vi "主画面.vi"() -> ()   [LabVIEW 2016]
uses:
  <vilib>/Utility/miscctls.llb/LVPointTypeDef.ctl
  <vilib>/Averna/Notify Icon/NotifyIcon.llb/BalloonIcon.ctl
  <vilib>/Utility/config.llb/Write Key (String).vi
  <vilib>/Utility/config.llb/Write Key (U32).vi
  <vilib>/Utility/config.llb/Read Key (String).vi
  <vilib>/Utility/config.llb/Read Key (I32).vi
  <vilib>/Averna/Notify Icon/NotifyIcon.llb/GetSelectedItemEvent.vi
  <vilib>/Averna/Notify Icon/NotifyIcon.llb/SetVisible.vi
  <vilib>/Averna/Notify Icon/NotifyIcon.llb/SetMenuDefaultItem.vi
  <vilib>/Averna/Notify Icon/NotifyIcon.llb/SetTipText.vi
  <vilib>/FTP/NI_FTP.lvlib
  <vilib>/Averna/Notify Icon/NotifyIcon.llb/NotifyIcon.lvclass
  <vilib>/Utility/config.llb/NI_LVConfig.lvlib
panel:
  in  "AniGIF":refnum<k7>(container)
  in  "TCP数据输入":string
  in  "开机启动":bool
  in  "超时毫秒(25000)":i32
  in  "模式（标准）":T1(ring)
  out "error out":errorcluster
  in  "停止":bool
  out "程序更新次数":i32
  out "错误TCP":errorcluster caption="错误输出"
  out "连接ID":refnum<k5>
  in  "远程端口或服务名称":u16=1000
  in  "地址":string="127.0.0.1"
  out "当前状态":enum16{"open", "read", "write", "close"}(ring)
  out "通讯":bool
  out "心跳包计数":i32
  out "TCP数据读取":string
  in  "流程启动":bool
  in  "QN":string
  out "日期/时间字符串":string
  out "步骤":string
  out "流程信息":string
  in  "local path":path=path "C:/Users/Administrator/Desktop/ftp接收文件/一体化微型水质监测站.exe"
  in  "filename":string="一体化微型水质监测站.exe"
  in  "passWord":string="std23506"
  in  "userName":string="cc"
  in  "address":string="192.168.16.237"
  # "examples:\nftp.ni.com\nftp.kernel.org\nftp.microsoft.com"
  # "从TCP端读取的信息有：\n1.FTP的address\n2.username\n3.password\n4.filename(.exe)\n5.local path"
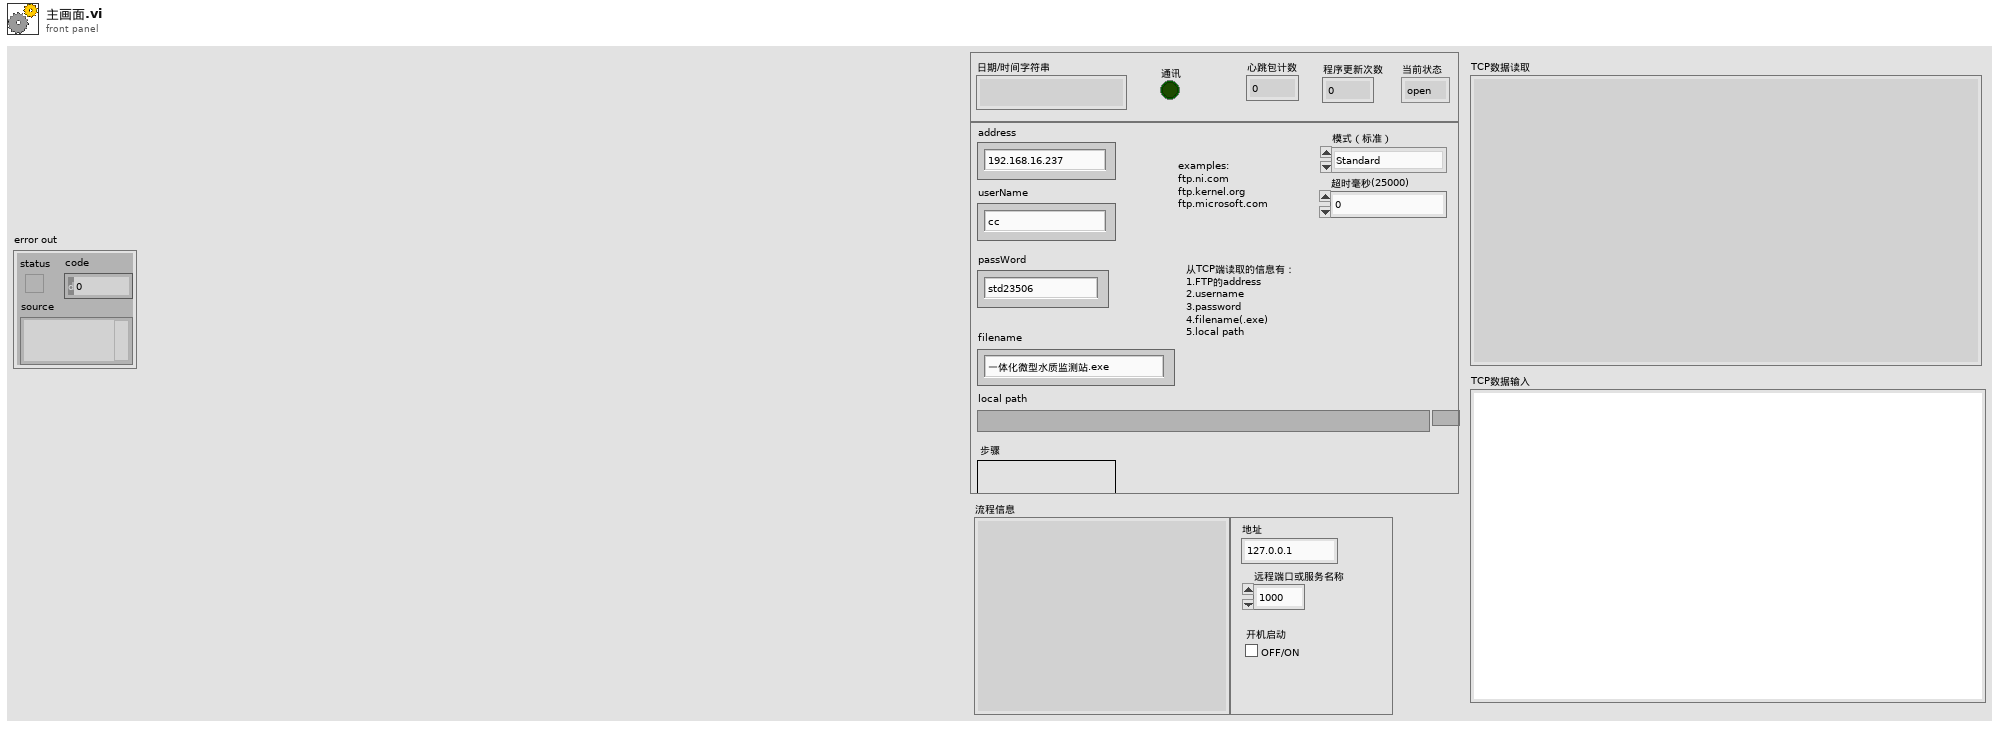
[diagram p1: front panel]
types:
  T1 = enum16{"Standard", "Buffered", "CRLF", "Immediate"}
  T2 = typedef "LVPointTypeDef.ctl" = cluster{"Horizontal":i16, "Vertical":i16}
  T3 = typedef "NI_LVConfig.lvlib/Config Data RefNum.ctl" = refnum<k1>
  T4 = enum32{"invalid app kind", "Development System", "Run Time System", "Student Edition", "Embedded LabVIEW", "Evaluation", "Custom"}
  T5 = enum32{"Invalid", "Standard", "Closed", "Hidden", "Minimized", "Maximized"}
  T6 = enum16{"init", "download", "close", "replace", "open", "over"}
  T7 = typedef "NotifyIcon.lvlib/NotifyIcon.lvclass/BalloonIcon.ctl" = enum32{"None", "Information", "Warning", "Error"}
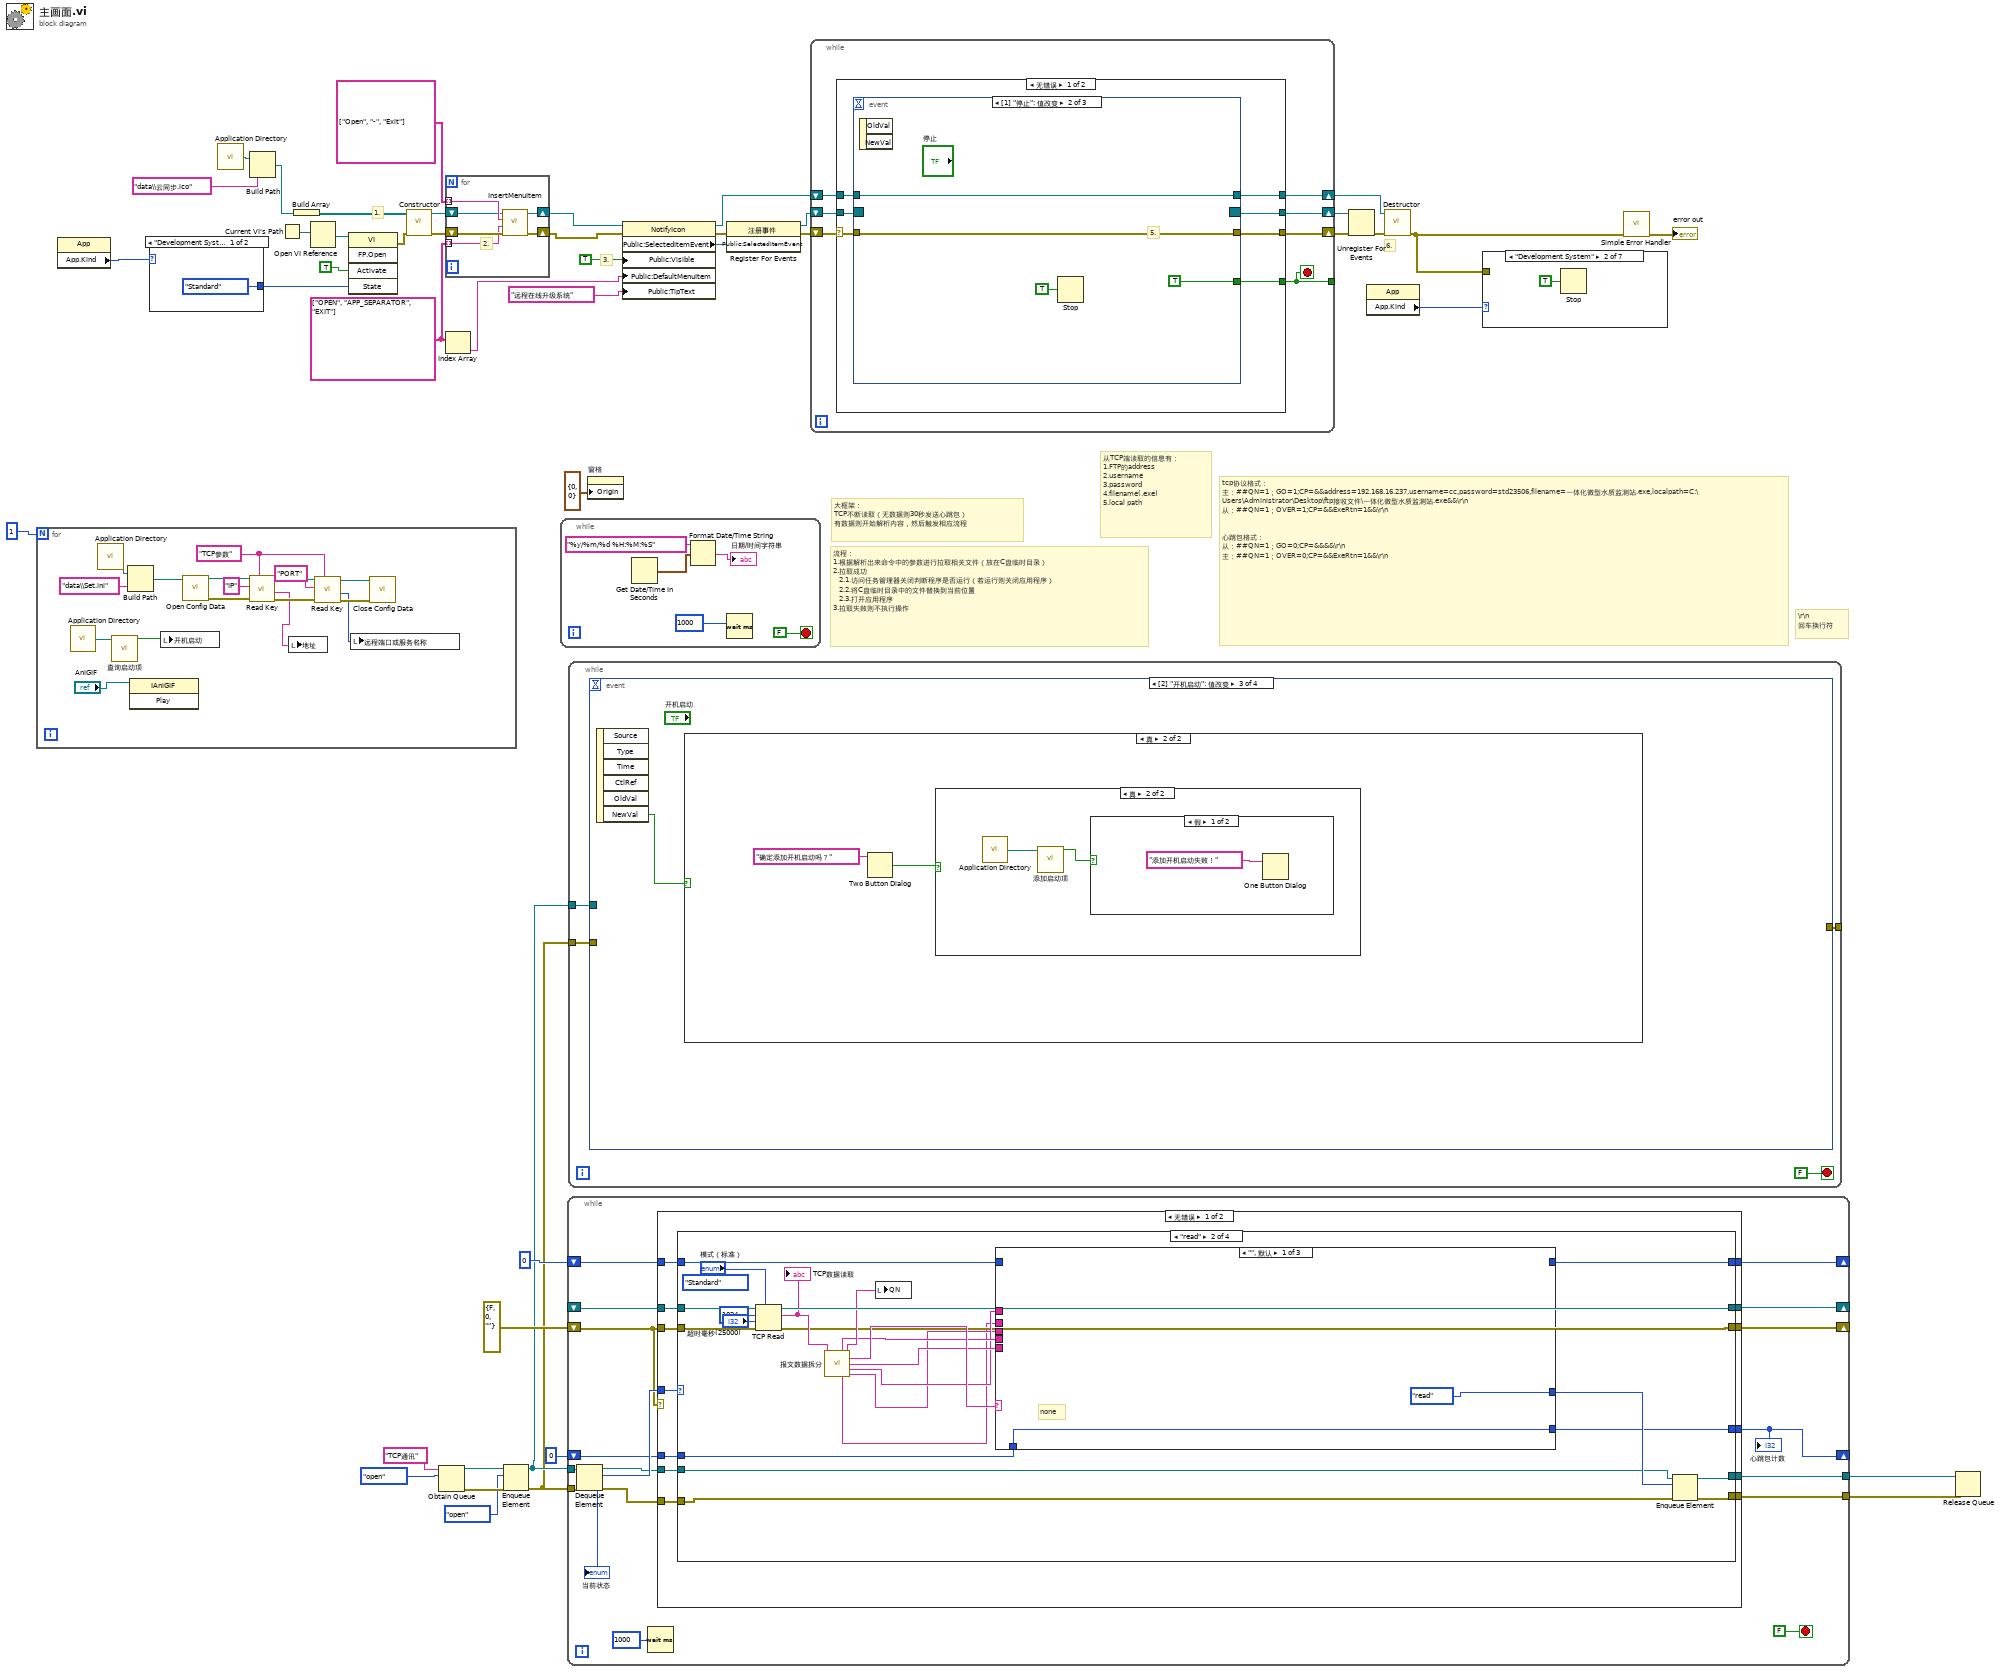
[diagram p0: block diagram]
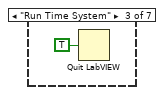
[diagram p3: hidden frame]
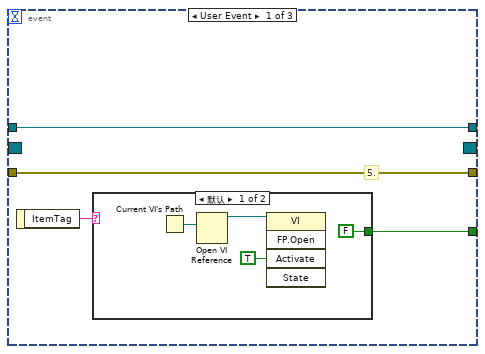
[diagram p8: hidden frame]
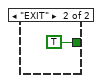
[diagram p9: hidden frame]
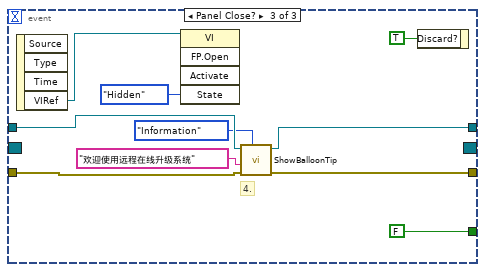
[diagram p10: hidden frame]
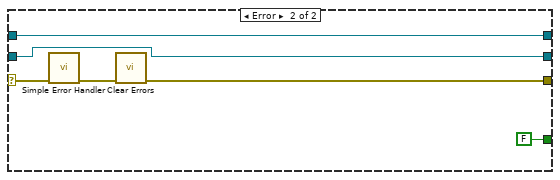
[diagram p11: hidden frame]
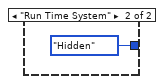
[diagram p12: hidden frame]
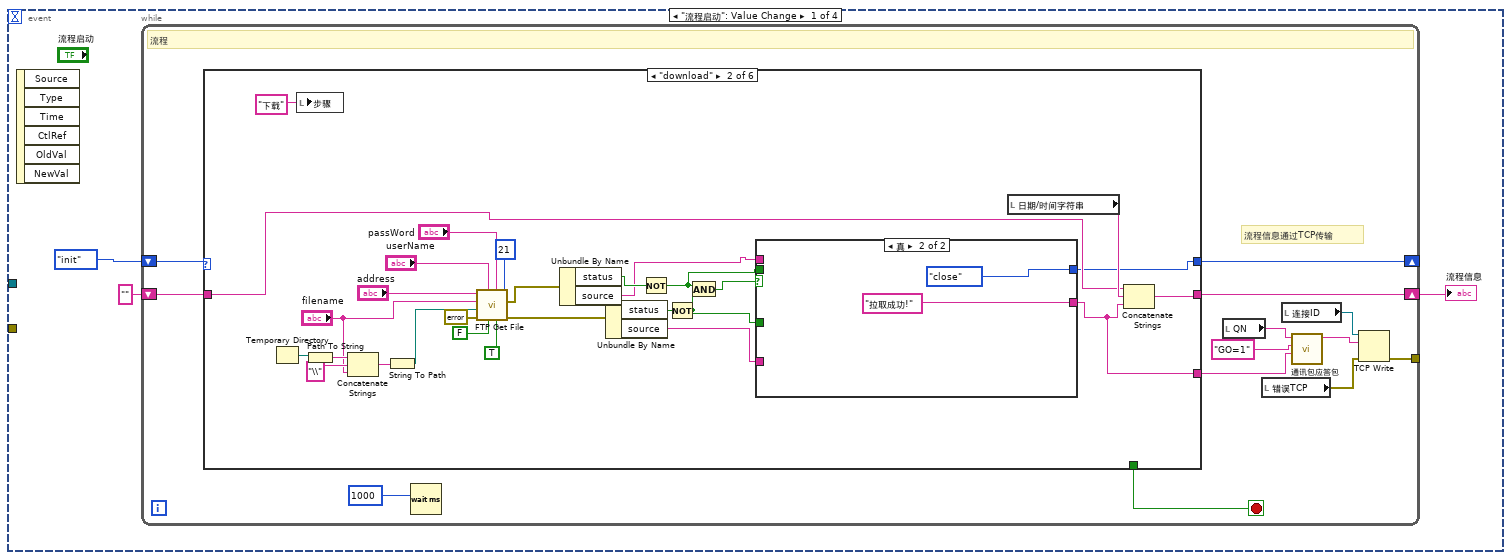
[diagram p13: hidden frame]
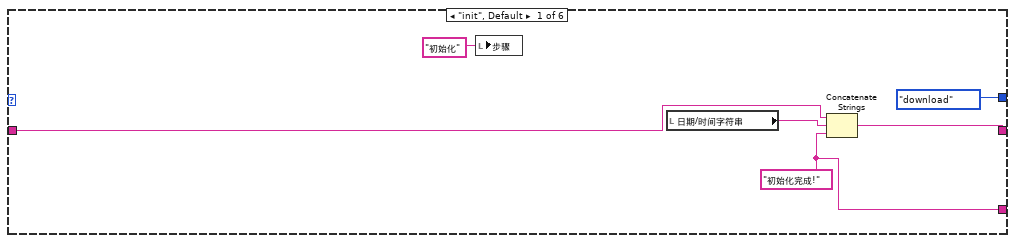
[diagram p14: hidden frame]
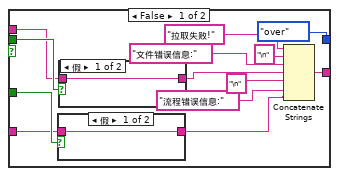
[diagram p15: hidden frame]
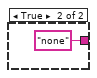
[diagram p16: hidden frame]
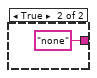
[diagram p17: hidden frame]
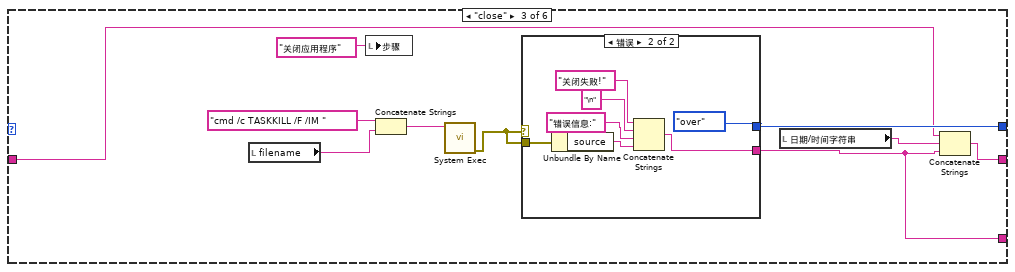
[diagram p18: hidden frame]
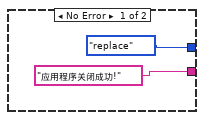
[diagram p19: hidden frame]
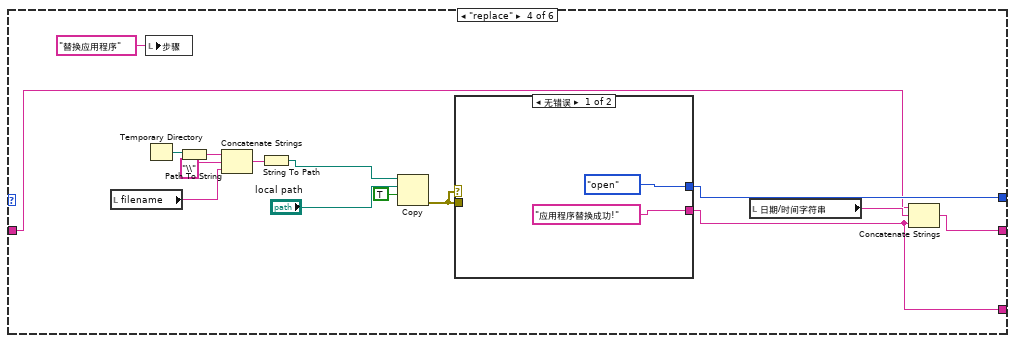
[diagram p20: hidden frame]
diagram:
  w24 = string[] ["OPEN", "APP_SEPARATOR", "EXIT"]
  # "6."
  # "3."
  # "1."
  # "\\r\\n\n回车换行符"
  # "tcp协议格式：\n主：##QN=1；GO=1;CP=&&address=192.168.16.237,username=cc,password=std23506,filename=一体化微型水质监测站.exe,localpath=C:\\Users\\Administrator\\Desktop\\ftp接收文件\\一体化微型水质监测站.exe&&\\r\\n\n从：##QN=1；OVER=1;CP=&&ExeRtn=1&&\\r\\n\n\n\n心跳包格式：\n从：##QN=1；GO=0;CP=&&&&\\r\\n\n主：##QN=1；OVER=0;CP=&&ExeRtn=1&&\\r\\n"
  # "从TCP端读取的信息有：\n1.FTP的address\n2.username\n3.password\n4.filename(.exe)\n5.local path"
  # "流程：\n1.根据解析出来命令中的参数进行拉取相关文件（放在C盘临时目录）\n2.拉取成功\n   2.1.访问任务管理器关闭判断程序是否运行（若运行则关闭应用程序）\n   2.2.将C盘临时目录中的文件替换到当前位置\n   2.3.打开应用程序\n3.拉取失败则不执行操作"
  # "大框架：\nTCP不断读取（无数据则30秒发送心跳包）\n有数据则开始解析内容，然后触发相应流程"
  n1 = for {
    N: 1 -> [_]
    w52 = "TCP参数" ("section")
    n2 = call <vilib>:"Application Directory.vi"() -> ("Application Directory"=w48:path)
    n3 = call <vilib>:"Application Directory.vi"() -> ("Application Directory"=w60:path)
    n4 = call "查询启动项.vi"("启动文件路径"=w48) -> ("包含启动项"=w47:bool)  [unwired: 9 in, 1 out]
    n5 = Build Path(base path=w60, name or relative path="data\\Set.ini" ("名称或相对路径")) -> (appended path=w58:path)
    n6 = invoke class="IAniGIF" method="Play"(reference="AniGIF") -> ()  [unwired: 2 in, 3 out]
    n7 = local write "开机启动"(w47) -> ()
    n8 = call <vilib>:"Open Config Data.vi"("configuration file path"=w58) -> ("error out"=w61:errorcluster, "refnum"=w62:T3)  [unwired: 8 in, 1 out]
    n9 = call-poly <vilib>:"Read Key.vi"("section"=w52, "error in (no error)"=w61, "key"="IP", "refnum"=w62) -> ("error out"=w56:errorcluster, "value"=w50:string, "refnum out"=w57:T3)  [unwired: 4 in, 1 out]
    n10 = local write "地址"(w50) -> ()
    n11 = call-poly <vilib>:"Read Key.vi"("section"=w52, "error in (no error)"=w56, "key"="PORT", "refnum"=w57) -> ("error out"=w54:errorcluster, "value"=w49:i32, "refnum out"=w55:T3)  [unwired: 4 in, 1 out]
    n12 = local write "远程端口或服务名称"(w49) -> ()
    n13 = call <vilib>:"Close Config Data.vi"("error in (no error)"=w54, "refnum"=w55) -> ()  [unwired: 8 in, 2 out]
  }
  n14 = property class="App"() -> ("App.Kind"=w32:T4)  [unwired: 2 in, 2 out]
  n15 = case shown="\"Development System\", 默认" w32 {
    tunnel: [T5."Standard" ("状态") T5."Hidden" ("状态")] -> w4
    frame "Development System", Default {
    }
    frame "Run Time System" {
    }
  }
  n16 = call <vilib>:"Application Directory.vi"() -> ("Application Directory"=w26:path)
  n17 = Build Path(base path=w26, name or relative path="data\\云同步.ico" ("名称或相对路径")) -> (appended path=w16:path)
  n18 = Current VI's Path() -> (path=w29:path)
  n19 = Build Array(w16) -> (w21:path[])
  n20 = Open VI Reference(vi path=w29) -> (vi reference=w30:refnum<vi>)  [unwired: 5 in, 1 out]
  n21 = invoke class="VI" method="FP.Open"(reference=w30, "Activate"=TRUE ("激活？"), "State"=w4) -> (error out=w31:errorcluster)  [unwired: 2 in, 4 out]
  n22 = call <vilib>:"Constructor.vi"("error in"=w31, "IconFilePathList"=w21) -> ("error out"=w17:errorcluster, "NotifyIcon"=w25:refnum<class "NotifyIcon.lvclass">)  [unwired: 8 in]
  n23 = Obtain Queue(name (unnamed)="TCP通讯" ("名称（未命名）"), element data type=enum16{"open", "read", "write", "close"}."open") -> (queue out=w39:refnum<queue>, error out=w38:errorcluster)  [unwired: 3 in, 1 out]
  n24 = for {
    shift-right: [w69] -> w2
    shift-left: w17 -> [w70]
    tunnel: string[] ["Open", "-", "Exit"] -> [w68] mode=indexing
    tunnel: w24 -> [w67] mode=indexing
    shift-right: [w65] -> w3
    shift-left: w25 -> [w66]
    # "2."
    n25 = call <vilib>:"InsertMenuItem.vi"("error in"=w70, "ItemTag"=w67, "ItemName"=w68, "NotifyIcon in"=w66) -> ("error out"=w69:errorcluster, "NotifyIcon out"=w65:refnum<class "NotifyIcon.lvclass">)  [unwired: 6 in]
  }
  n26 = Index Array(array=w24) -> (element=w23:string)  [unwired: 1 in]
  n27 = Enqueue Element(queue=w39, element=enum16{"open", "read", "write", "close"}."open" ("元素"), error in (no error)=w38) -> (queue out=w34:refnum<queue>, error out=w33:errorcluster)  [unwired: 1 in, 1 out]
  n28 = while {
    stop <- FALSE stop-if-true
    n29 = Get Date/Time In Seconds() -> (seconds since 1Jan1904=w71:timestamp)
    n30 = Format Date/Time String(time format string (%c)="%y/%m/%d %H:%M:%S" ("时间格式字符串(%c)"), seconds (now)=w71) -> (date/time string=→"日期/时间字符串":string)  [unwired: 1 in]
    n31 = Wait (ms)(milliseconds to wait=u32 1000 ("等待时间（毫秒）")) -> ()  [unwired: 1 out]
  }
  n32 = while {
    shift-right: [w90] -> _
    shift-left: _ -> [w89]
    shift-right: [w76] -> _
    shift-left: errorcluster {"status"=FALSE, "code"=0, "source"=""} ("error out") -> [w79]
    tunnel: w34 -> [w88]
    tunnel: w33 -> [w87]
    tunnel: [w85] -> w43
    tunnel: [w84] -> w42
    shift-right: [w80] -> _
    shift-left: 0 -> [w81]
    shift-right: [w77] -> _
    shift-left: 0 -> [w78]
    stop <- FALSE stop-if-true
    n33 = Dequeue Element(queue=w88, error in (no error)=w87) -> (queue out=w82:refnum<queue>, element=w86:enum16{"open", "read", "write", "close"}, error out=w83:errorcluster)  [unwired: 1 in, 1 out]
    "当前状态" <- w86
    n34 = Wait (ms)(milliseconds to wait=u32 1000 ("等待时间（毫秒）")) -> ()  [unwired: 1 out]
    n35 = case shown="无错误" w79 {
      selector: w79 -> [_ w200]
      tunnel: [w105 w196] -> w90
      tunnel: w89 -> [w104 w198]
      tunnel: w79 -> [w103 w197]
      tunnel: w86 -> [w102 _]
      tunnel: [w101 w192] -> w85
      tunnel: [w100 w191] -> w84
      tunnel: w83 -> [w99 w193]
      tunnel: w82 -> [w98 w194]
      tunnel: w81 -> [w97 _]
      tunnel: [w96 _] -> w80
      tunnel: [w95 w195] -> w76
      tunnel: w78 -> [w94 _]
      tunnel: [w93 _] -> w77
      frame No Error {
        n36 = case shown="\"read\"" w102 {
          tunnel: [w116 w138 w179 w188] -> w105
          tunnel: [w106 w122 w178 w187] -> w95
          tunnel: w104 -> [_ w140 w181 w190]
          tunnel: w103 -> [_ w139 w180 w189]
          tunnel: [w115 w131 w174 w183] -> w101
          tunnel: [w114 w130 w173 w182] -> w100
          tunnel: w99 -> [w112 w132 w176 w184]
          tunnel: w98 -> [w111 w133 w177 w185]
          tunnel: w97 -> [_ w129 _ _]
          tunnel: [_ w128 _ _] -> w96
          tunnel: w94 -> [_ w121 _ _]
          tunnel: [_ w120 _ _] -> w93
          frame "open", Default {
            (unwired) u16 1000 ("远程端口或服务名称")
            (unwired) "127.0.0.1" ("地址")
            n37 = TCP Open Connection(address="地址", remote port or service name="远程端口或服务名称") -> (connection ID=w116:refnum<k5>, error out=w106:errorcluster)  [unwired: 3 in]
            "连接ID" <- w116
            "错误TCP" <- w106
            n38 = Unbundle By Name(w106) -> ("status"=w107:bool)
            n39 = Not(x=w107) -> (.not. x?=→"通讯":bool)
            n40 = Enqueue Element(queue=w111, element=enum16{"open", "read", "write", "close"}."read", error in (no error)=w112) -> (queue out=w115:refnum<queue>, error out=w114:errorcluster)  [unwired: 1 in, 1 out]
          }
          frame "read" {
            (unwired) T1."Standard" ("模式（标准）")
            n41 = TCP Read(connection ID=w140, bytes to read=1024 ("读取的字节"), error in (no error)=w139, 7:"模式（标准）", 9:"超时毫秒(25000)") -> (connection ID out=w138:refnum<k5>, data out=w137:string, error out=w122:errorcluster)
            "TCP数据读取" <- w137
            n42 = call "报文数据拆分.vi"("字符串"=w137) -> ("filename"=w127:string, "QN"=w135:string, "GO"=w136:string, "address"=w126:string, "username"=w125:string, "localpath"=w119:string, "password"=w124:string)  [unwired: 8 in]
            n43 = local write "QN"(w135) -> ()
            n44 = case shown="\"\", 默认" w136 {
              tunnel: [enum16{"open", "read", "write", "close"}."read" w147 w162] -> w134
              tunnel: w129 -> [w141 w146 w163]
              tunnel: [w141 w145 w163] -> w128
              tunnel: w127 -> [_ _ w161]
              tunnel: w126 -> [_ _ w160]
              tunnel: w125 -> [_ _ w159]
              tunnel: w124 -> [_ _ w158]
              tunnel: w121 -> [_ _ w157]
              tunnel: [_ _ w156] -> w120
              tunnel: w119 -> [_ _ w154]
              frame "", Default {
                # "none"
              }
              frame "0" {
                # "心跳包"
                n45 = Increment(x=w146) -> (x+1=w145:i32)
                n46 = Greater Or Equal?(x=w145, y=30) -> (x >= y?=w143:bool)
                n47 = case shown="真" w143 {
                  tunnel: [enum16{"open", "read", "write", "close"}."read" enum16{"open", "read", "write", "close"}."write"] -> w147
                  frame False {
                  }
                  frame True {
                    # "心跳包"
                    n48 = call "通讯包应答包.vi"("数据字段"="" ("GO/OVER"), "GO/OVER"="GO=0", "QN"="1") -> ("通讯包字符串"=w152:string)  [unwired: 8 in]
                    n49 = local write "TCP数据输入"(w152) -> ()
                  }
                }
              }
              frame "1" {
                # "流程启动"
                n50 = flat-sequence {
                  tunnel: [enum16{"open", "read", "write", "close"}."read"] -> w162
                  frame #0 {
                    n51 = property on="流程启动" class="Bool (严格)"("Val(Sgnl)"=TRUE) -> ()  [unwired: 2 in, 2 out]
                  }
                  frame #1 {
                    n52 = Wait (ms)(milliseconds to wait=u32 500 ("等待时间（毫秒）")) -> ()  [unwired: 1 out]
                  }
                  frame #2 {
                    n53 = property on="流程启动" class="Bool (严格)"("Value"=FALSE) -> ()  [unwired: 2 in, 2 out]
                  }
                  frame #3 {
                    n54 = disable-structure shown="禁用" {
                      frame Disabled {
                        # "应答"
                        n55 = call "通讯包应答包.vi"("数据字段"="ExeRtn=1" ("GO/OVER"), "GO/OVER"="OVER=1", "QN"="QN") -> ("通讯包字符串"=w167:string)  [unwired: 8 in]
                        n56 = local write "TCP数据输入"(w167) -> ()
                      }
                      frame Enabled {
                      }
                    }
                  }
                  frame #4 {
                  }
                }
                n57 = local write "filename"(w161) -> ()
                n58 = local write "address"(w160) -> ()
                n59 = local write "userName"(w159) -> ()
                n60 = local write "passWord"(w158) -> ()
                n61 = String To Path(string=w154) -> (path=w155:path)
                n62 = Increment(x=w157) -> (x+1=w156:i32)
                "程序更新次数" <- w156
                n63 = local write "local path"(w155) -> ()
              }
            }
            n64 = Enqueue Element(queue=w133, element=w134, error in (no error)=w132) -> (queue out=w131:refnum<queue>, error out=w130:errorcluster)  [unwired: 1 in, 1 out]
          }
          frame "write" {
            n65 = TCP Write(connection ID=w181, data in="TCP数据输入", error in (no error)=w180) -> (connection ID out=w179:refnum<k5>, error out=w178:errorcluster)  [unwired: 1 in, 1 out]
            n66 = Enqueue Element(queue=w177, element=enum16{"open", "read", "write", "close"}."read", error in (no error)=w176) -> (queue out=w174:refnum<queue>, error out=w173:errorcluster)  [unwired: 1 in, 1 out]
          }
          frame "close" {
            n67 = TCP Close Connection(connection ID=w190, error in (no error)=w189) -> (connection ID out=w188:refnum<k5>, error out=w187:errorcluster)  [unwired: 1 in]
            n68 = Enqueue Element(queue=w185, element=enum16{"open", "read", "write", "close"}."open", error in (no error)=w184) -> (queue out=w183:refnum<queue>, error out=w182:errorcluster)  [unwired: 1 in, 1 out]
          }
        }
      }
      frame Error {
        n69 = Unbundle By Name(w200) -> ("code"=w199:i32)
        n70 = case shown="63, 66" w199 {
          tunnel: w198 -> [w208 w214 w219]
          tunnel: w197 -> [w207 w215 w218]
          tunnel: [w208 w214 w219] -> w196
          tunnel: [w201 w213 w217] -> w195
          tunnel: w194 -> [w205 w212 w223]
          tunnel: w193 -> [w204 w211 w222]
          tunnel: [w203 w209 w221] -> w192
          tunnel: [w202 w210 w220] -> w191
          frame 0, Default {
            n71 = call <vilib>:"Clear Errors.vi"("error in (no error)"=w207) -> ("error out"=w201:errorcluster)  [unwired: 5 in, 1 out]
            n72 = Enqueue Element(queue=w205, element=enum16{"open", "read", "write", "close"}."read" ("元素"), error in (no error)=w204) -> (queue out=w203:refnum<queue>, error out=w202:errorcluster)  [unwired: 1 in, 1 out]
          }
          frame 1 {
            n73 = call <vilib>:"Clear Errors.vi"("error in (no error)"=w215) -> ("error out"=w213:errorcluster)  [unwired: 5 in, 1 out]
            n74 = Enqueue Element(queue=w212, element=enum16{"open", "read", "write", "close"}."open" ("元素"), error in (no error)=w211) -> (queue out=w209:refnum<queue>, error out=w210:errorcluster)  [unwired: 1 in, 1 out]
          }
          frame 63, 66 {
            n75 = call <vilib>:"Clear Errors.vi"("error in (no error)"=w218) -> ("error out"=w217:errorcluster)  [unwired: 5 in, 1 out]
            n76 = Enqueue Element(queue=w223, element=enum16{"open", "read", "write", "close"}."close" ("元素"), error in (no error)=w222) -> (queue out=w221:refnum<queue>, error out=w220:errorcluster)  [unwired: 1 in, 1 out]
          }
        }
      }
    }
    "心跳包计数" <- w80
  }
  n77 = while {
    tunnel: w34 -> [w227]
    tunnel: w33 -> [w226]
    tunnel: [w225] -> _
    stop <- FALSE stop-if-true
    n78 = event shown="[2] \"开机启动\": 值改变" {
      selector: _ -> [_ _ _ _]
      dyn-events: _ -> [_ _ _ _]
      timeout: _ -> [_ _ _ _]
      tunnel: w227 -> [_ w386 _ _]
      tunnel: w226 -> [_ w385 _ _]
      tunnel: [_ w384 _ _] -> w225
      event "流程启动": Value Change {
        n79 = event-data() -> ()  [unwired: 1 in, 6 out]
        n80 = while "While循环" {
          shift-right: [w232] -> _
          shift-left: T6."init" -> [w233]
          shift-right: [w240] -> w229
          shift-left: "" -> [w242]
          tunnel: [w236] -> _
          stop <- w243 stop-if-true
          # "流程信息通过TCP传输"
          # "流程"
          n81 = case shown="\"download\"" w233 {
            tunnel: [T6."download" w262 w304 w320 w344 T6."over"] -> w232
            tunnel: [w249 w261 w300 w322 w343 w360] -> w240
            tunnel: [_ _ _ _ _ TRUE] -> w243
            tunnel: w242 -> [w248 w263 w299 w318 w342 w363]
            tunnel: [w246 w260 w298 w321 w341 "更新完成!" ("步骤")] -> w235
            frame "init", Default {
              w246 = "初始化完成!" ("字符串")
              n82 = local write "步骤"("初始化" ("步骤")) -> ()
              n83 = local read "日期/时间字符串"() -> (w247:string)
              n84 = Concatenate Strings(w248, w247, w246) -> (w249:string)
            }
            frame "download" {
              n85 = Temporary Directory() -> (w259:path)
              n86 = local write "步骤"("下载" ("步骤")) -> ()
              n87 = Path To String(path=w259) -> (string=w258:string)
              n88 = Concatenate Strings(w258, "\\" ("字符串"), "filename") -> (w255:string)
              n89 = String To Path(string=w255) -> (path=w254:path)
              n90 = call <vilib>:"FTP Get File.vi"("remote port (21)"=u16 21, "active (T)"=TRUE, "password"="passWord", "binary (F)"=FALSE, "user"="userName", "error in (no error)"=errorcluster {"status"=FALSE, "code"=0, "source"=""}, "local path"=w254, "remote path"="filename", "host"="address") -> ("error out"=w274:errorcluster, "file error"=w275:errorcluster)  [unwired: 1 in]
              n91 = Unbundle By Name(w275) -> ("status"=w276:bool, "source"=w273:string)
              n92 = Unbundle By Name(w274) -> ("status"=w277:bool, "source"=w271:string)
              n93 = Not(x=w276) -> (.not. x?=w272:bool)
              n94 = Not(x=w277) -> (.not. x?=w269:bool)
              n95 = And(x=w272, y=w269) -> (x .and. y?=w270:bool)
              n96 = case shown="真" w270 {
                tunnel: w272 -> [w291 _]
                tunnel: w273 -> [w290 _]
                tunnel: w269 -> [w287 _]
                tunnel: w271 -> [w286 _]
                tunnel: [w280 "拉取成功!" ("消息")] -> w260
                tunnel: [T6."over" T6."close"] -> w262
                frame False {
                  n97 = case shown="假" w287 {
                    tunnel: w286 -> [w292 _]
                    tunnel: [w292 "none" ("source")] -> w283
                    frame False {
                    }
                    frame True {
                    }
                  }
                  n98 = case shown="假" w291 {
                    tunnel: w290 -> [w294 _]
                    tunnel: [w294 "none" ("source")] -> w288
                    frame False {
                    }
                    frame True {
                    }
                  }
                  n99 = Concatenate Strings("拉取失败!" ("消息"), "\n" ("字符串"), "文件错误信息:" ("字符串"), w288, "\n" ("字符串"), "流程错误信息:" ("字符串"), w283) -> (w280:string)
                }
                frame True {
                }
              }
              n100 = local read "日期/时间字符串"() -> (w268:string)
              n101 = Concatenate Strings(w263, w268, w260) -> (w261:string)
            }
            frame "close" {
              n102 = local read "filename"() -> (w307:string)
              n103 = local write "步骤"("关闭应用程序" ("步骤")) -> ()
              n104 = Concatenate Strings("cmd /c TASKKILL /F /IM " ("command line"), w307) -> (w306:string)
              n105 = call <vilib>:"System Exec.vi"("command line"=w306) -> ("error out"=w302:errorcluster)  [unwired: 7 in, 3 out]
              n106 = case shown="错误" w302 {
                tunnel: [T6."replace" T6."over"] -> w304
                tunnel: w302 -> [_ w316]
                tunnel: ["应用程序关闭成功!" ("步骤") w311] -> w298
                frame No Error {
                }
                frame Error {
                  n107 = Unbundle By Name(w316) -> ("source"=w315:string)
                  n108 = Concatenate Strings("关闭失败!" ("消息"), "\n" ("字符串"), "错误信息:" ("字符串"), w315) -> (w311:string)
                }
              }
              n109 = local read "日期/时间字符串"() -> (w301:string)
              n110 = Concatenate Strings(w299, w301, w298) -> (w300:string)
            }
            frame "replace" {
              n111 = local read "filename"() -> (w323:string)
              n112 = local write "步骤"("替换应用程序" ("步骤")) -> ()
              n113 = Temporary Directory() -> (w328:path)
              n114 = Path To String(path=w328) -> (string=w327:string)
              n115 = Concatenate Strings(w327, "\\" ("字符串"), w323) -> (w325:string)
              n116 = String To Path(string=w325) -> (path=w324:path)
              n117 = Copy(9:TRUE ("覆盖(F)"), 10:"local path", 11:w324) -> (0:w317:errorcluster)  [unwired: 2 in, 2 out]
              n118 = case shown="无错误" w317 {
                tunnel: [T6."open" T6."over"] -> w320
                tunnel: w317 -> [_ w340]
                tunnel: ["应用程序替换成功!" ("步骤") w335] -> w321
                frame No Error {
                }
                frame Error {
                  n119 = Unbundle By Name(w340) -> ("source"=w339:string)
                  n120 = Concatenate Strings("替换失败!" ("消息"), "\n" ("字符串"), "错误信息:" ("字符串"), w339) -> (w335:string)
                }
              }
              n121 = local read "日期/时间字符串"() -> (w319:string)
              n122 = Concatenate Strings(w318, w319, w321) -> (w322:string)
            }
            frame "open" {
              n123 = local read "local path"() -> (w348:path)
              n124 = local write "步骤"("打开应用程序" ("步骤")) -> ()
              n125 = Path To String(path=w348) -> (string=w349:string)
              n126 = call <vilib>:"System Exec.vi"("wait until completion? (T)"=FALSE, "command line"=w349) -> ("error out"=w346:errorcluster)  [unwired: 6 in, 3 out]
              n127 = case shown="错误" w346 {
                tunnel: [T6."over" T6."over"] -> w344
                tunnel: w346 -> [_ w359]
                tunnel: ["应用程序打开成功!" ("步骤") w354] -> w341
                frame No Error {
                }
                frame Error {
                  n128 = Unbundle By Name(w359) -> ("source"=w358:string)
                  n129 = Concatenate Strings("打开失败!" ("消息"), "\n" ("字符串"), "错误信息:" ("字符串"), w358) -> (w354:string)
                }
              }
              n130 = local read "日期/时间字符串"() -> (w345:string)
              n131 = Concatenate Strings(w342, w345, w341) -> (w343:string)
            }
            frame "over" {
              n132 = Build Array(w363) -> (w365:string[])
              n133 = call "发送数据记录到文档(子VI).vi"("数组"=w365) -> ("错误输出"=w364:errorcluster)  [unwired: 9 in]
              n134 = case shown="无错误" w364 {
                tunnel: w363 -> [w368 w369]
                tunnel: [w368 w369] -> w360
                frame No Error {
                }
                frame Error {
                }
              }
              n135 = local write "步骤"("更新完成" ("步骤")) -> ()
            }
          }
          n136 = Wait (ms)(milliseconds to wait=u32 1000 ("等待时间（毫秒）")) -> ()  [unwired: 1 out]
          n137 = local read "QN"() -> (w234:string)
          n138 = local read "错误TCP"() -> (w237:errorcluster)
          n139 = local read "连接ID"() -> (w239:refnum<k5>)
          n140 = call "通讯包应答包.vi"("数据字段"=w235, "GO/OVER"="GO=1", "QN"=w234) -> ("通讯包字符串"=w238:string)  [unwired: 8 in]
          n141 = TCP Write(connection ID=w239, data in=w238, error in (no error)=w237) -> (error out=w236:errorcluster)  [unwired: 1 in, 2 out]
        }
        "流程信息" <- w229
      }
      event "地址", "远程端口或服务名称": Value Change {
        w378 = "TCP参数" ("section")
        n142 = event-data() -> ()  [unwired: 1 in, 6 out]
        n143 = call <vilib>:"Application Directory.vi"() -> ("Application Directory"=w382:path)
        n144 = Build Path(base path=w382, name or relative path="data\\Set.ini" ("名称或相对路径")) -> (appended path=w380:path)
        n145 = call <vilib>:"Open Config Data.vi"("configuration file path"=w380) -> ("error out"=w379:errorcluster, "refnum"=w383:T3)  [unwired: 8 in, 1 out]
        n146 = local read "地址"() -> (w371:string)
        n147 = local read "远程端口或服务名称"() -> (w370:u16)
        n148 = call-poly <vilib>:"Write Key.vi"("section"=w378, "error in (no error)"=w379, "value"=w371, "key"="IP", "refnum"=w383) -> ("error out"=w375:errorcluster, "refnum out"=w376:T3)  [unwired: 4 in, 1 out]
        n149 = call-poly <vilib>:"Write Key.vi"("section"=w378, "error in (no error)"=w375, "value"=w370, "key"="PORT", "refnum"=w376) -> ("error out"=w374:errorcluster, "refnum out"=w377:T3)  [unwired: 4 in, 1 out]
        n150 = call <vilib>:"Close Config Data.vi"("error in (no error)"=w374, "refnum"=w377) -> ()  [unwired: 8 in, 2 out]
        n151 = Enqueue Element(queue=w386, element=enum16{"open", "read", "write", "close"}."close", error in (no error)=w385) -> (error out=w384:errorcluster)  [unwired: 1 in, 2 out]
      }
      event "开机启动": Value Change {
        n152 = event-data() -> ("NewVal"=w388:bool)  [unwired: 1 in, 5 out]
        n153 = case shown="真" w388 {
          frame False {
            n154 = Two Button Dialog(message="确定删除开机启动吗？" ("消息")) -> (T button?=w389:bool)  [unwired: 2 in]
            n155 = case shown="真" w389 {
              frame False {
              }
              frame True {
                n156 = call <vilib>:"Application Directory.vi"() -> ("Application Directory"=w392:path)
                n157 = call "删除启动项.vi"("启动文件路径"=w392) -> ("删除标记"=w391:bool)  [unwired: 9 in, 1 out]
                n158 = case shown="真" w391 {
                  frame False {
                    n159 = One Button Dialog(message="删除开机启动失败！" ("消息")) -> ()  [unwired: 1 in, 1 out]
                  }
                  frame True {
                    n160 = One Button Dialog(message="删除开机启动成功！" ("消息")) -> ()  [unwired: 1 in, 1 out]
                  }
                }
              }
            }
          }
          frame True {
            n161 = Two Button Dialog(message="确定添加开机启动吗？" ("消息")) -> (T button?=w395:bool)  [unwired: 2 in]
            n162 = case shown="真" w395 {
              frame False {
              }
              frame True {
                n163 = call <vilib>:"Application Directory.vi"() -> ("Application Directory"=w398:path)
                n164 = call "添加启动项.vi"("启动文件路径"=w398) -> ("添加成功标记"=w397:bool)  [unwired: 9 in, 1 out]
                n165 = case shown="假" w397 {
                  frame False {
                    n166 = One Button Dialog(message="添加开机启动失败！" ("消息")) -> ()  [unwired: 1 in, 1 out]
                  }
                  frame True {
                    n167 = One Button Dialog(message="添加开机启动成功！" ("消息")) -> ()  [unwired: 1 in, 1 out]
                  }
                }
              }
            }
          }
        }
      }
      event Timeout {
        n168 = event-data() -> ()  [unwired: 1 in, 3 out]
      }
    }
  }
  n169 = property on="窗格" class="Pane"("Origin"=T2 {"Horizontal"=0, "Vertical"=0} ("原点")) -> ()  [unwired: 2 in, 2 out]
  n170 = property class="NotifyIcon"(reference=w3, error in=w2, "Public:Visible"=TRUE ("Visible"), "Public:DefaultMenuItem"=w23, "Public:TipText"="远程在线升级系统" ("TipText")) -> (reference out=w8:refnum<class "NotifyIcon.lvclass">, error out=w18:errorcluster, "Public:SelectedItemEvent"=w19:refnum<user-event>)
  n171 = register-events(error in=w18, w19) -> (reference out=w7:refnum<event-registration>, error out=w6:errorcluster)  [unwired: 1 in]
  n172 = while {
    shift-right: [w404] -> w10
    shift-left: w6 -> [w403]
    shift-right: [w405] -> w13
    shift-left: w8 -> [w406]
    shift-right: [w402] -> w12
    shift-left: w7 -> [w407]
    tunnel: [w401] -> _
    stop <- w401 stop-if-true
    n173 = case shown="无错误" w403 {
      selector: w403 -> [w409 w443]
      tunnel: w407 -> [w414 w438]
      tunnel: w406 -> [w413 w439]
      tunnel: [w412 w439] -> w405
      tunnel: [w411 w441] -> w404
      tunnel: [w410 FALSE ("Discard?")] -> w401
      tunnel: [w408 w438] -> w402
      frame No Error {
        n174 = event shown="[1] \"停止\": 值改变" {
          selector: w414 -> [_ _ _]
          dyn-events: [_ _ _] -> w408
          timeout: _ -> [_ _ _]
          tunnel: w409 -> [w417 w427 w436]
          tunnel: [w417 w427 w435] -> w411
          tunnel: [w416 TRUE FALSE ("Discard?")] -> w410
          tunnel: w413 -> [w415 w425 w437]
          tunnel: [w415 w425 w434] -> w412
          event User Event {
            # "5."
            n175 = event-data() -> ("ItemTag"=w418:string)  [unwired: 1 in]
            n176 = case shown="默认" w418 {
              tunnel: [FALSE TRUE] -> w416
              frame Default {
                n177 = Current VI's Path() -> (path=w419:path)
                n178 = Open VI Reference(vi path=w419) -> (vi reference=w420:refnum<vi>)  [unwired: 5 in, 1 out]
                n179 = invoke class="VI" method="FP.Open"(reference=w420, "Activate"=TRUE ("激活？")) -> ()  [unwired: 3 in, 5 out]
              }
              frame "EXIT" {
              }
            }
          }
          event "停止": Value Change {
            # "5."
            n180 = event-data() -> ()  [unwired: 1 in, 2 out]
            n181 = Stop(stop? (T)=TRUE ("可见")) -> ()
          }
          event Panel Close? {
            # "4."
            n182 = event-data() -> ("VIRef"=w430:refnum<vi>)  [unwired: 1 in, 3 out]
            n183 = invoke class="VI" method="FP.Open"(reference=w430, "State"=T5."Hidden" ("状态")) -> ()  [unwired: 3 in, 5 out]
            n184 = call <vilib>:"ShowBalloonTip.vi"("Balloon Icon"=BalloonIcon."Information", "error in"=w436, "Text"="欢迎使用远程在线升级系统", "NotifyIcon in"=w437) -> ("error out"=w435:errorcluster, "NotifyIcon out"=w434:refnum<class "NotifyIcon.lvclass">)  [unwired: 6 in]
            n185 = event-data("Discard?"=TRUE ("放弃？")) -> ()  [unwired: 1 in, 1 out]
          }
        }
      }
      frame Error {
        n186 = call <vilib>:"Simple Error Handler.vi"("error in (no error)"=w443) -> ("error out"=w442:errorcluster)  [unwired: 4 in, 4 out]
        n187 = call <vilib>:"Clear Errors.vi"("error in (no error)"=w442) -> ("error out"=w441:errorcluster)  [unwired: 5 in, 1 out]
      }
    }
  }
  n188 = Unregister For Events(event registration refnum=w12, error in=w10) -> (error out=w9:errorcluster)
  n189 = property class="App"() -> ("App.Kind"=w14:T4)  [unwired: 2 in, 2 out]
  n190 = call <vilib>:"Destructor.vi"("error in"=w9, "NotifyIcon"=w13) -> ("error out"=w15:errorcluster)  [unwired: 9 in]
  n191 = case shown="\"Development System\"" w14 {
    tunnel: w15 -> [_ _ _ _ _ _ _]
    frame "invalid app kind", Default {
    }
    frame "Development System" {
      n192 = Stop(stop? (T)=TRUE ("可见")) -> ()
    }
    frame "Run Time System" {
      n193 = Quit LabVIEW(quit? (T)=TRUE ("退出？(T)")) -> ()
    }
    frame "Student Edition" {
    }
    frame "Embedded LabVIEW" {
    }
    frame "Evaluation" {
    }
    frame "Custom" {
    }
  }
  n194 = call <vilib>:"Simple Error Handler.vi"("error in (no error)"=w15) -> ("error out"=→"error out":errorcluster)  [unwired: 4 in, 4 out]
  n195 = Release Queue(queue=w43, error in (no error)=w42) -> ()  [unwired: 1 in, 3 out]
